vi "Load Project.vi"(8 "error in (no error)":errorcluster, 10 "Application in":refnum<data-value>, 11 "Plugin in":refnum<class "Plugin.lvclass">) -> (0 "error out":errorcluster, 1 "Succeed":bool, 2 "Application out":refnum<data-value>, 3 "Plugin out":refnum<class "Plugin.lvclass">)   [LabVIEW 2015, in "Plugin.lvclass"]
uses:
  Plugin.lvclass
  Application.lvclass
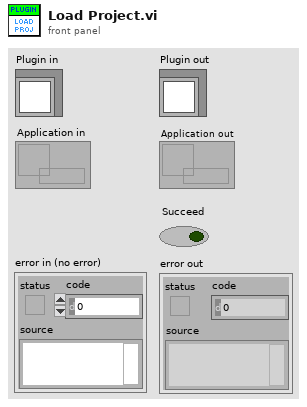
[diagram p1: front panel]
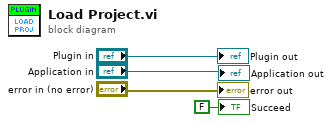
[diagram p0: block diagram]
diagram:
  "error out" <- "error in (no error)"
  "Plugin out" <- "Plugin in"
  "Application out" <- "Application in"
  "Succeed" <- FALSE ("Succeed")
